vi "Main.vi"() -> ()   [LabVIEW 2013]
doc: "This sample project is built upon the standard state machine template and shows how you could create an application that acquires, analyzes, and presents data. It includes functionality for presenting configuration dialogs, preserving settings between executions, loading and saving data, as well as exporting graph images and text files.\n\nIt is most appropriate for data that is acquired instantly as it does not allow for screen updates mid acquisition nor does it allow for continuous streaming to disk."
uses:
  TimeTagLV.lvlib
panel:
  in  "Record data":bool
  out "Initial time":dbl
  out "Elapsed time (s)":dbl
  out "FPGA_Run Status":dbl
  out "USB_Open Status":dbl
  out "Channel 4 Total\nCounts":dbl
  out "Channel 3 Total\nCounts":dbl
  out "Channel 2 Total\nCounts":dbl
  out "Channel 1 Total\nCounts":dbl
  in  "File Name":string
  out "?":dbl
  out "?":dbl
  out "?":dbl
  out "?":dbl
  in  "Runs":dbl
  out "stats":i32[](array[numeric])
  in  "stop":bool
  out "Channel 4 CPS":dbl(knob) scale=0.0..10000.0
  out "Channel 3 CPS":dbl(knob) scale=0.0..10000.0
  out "Channel 2 CPS":dbl(knob) scale=0.0..10000.0
  out "Channel 1 CPS":dbl(knob) scale=0.0..10000.0
  # "Channel 1"
  # "Channel 2"
  # "Channel 3"
  # "Channel 4"
  # "Coincidence Channels 1 & 2"
  # "Coincidence Channels 1 & 3"
  # "Coincidence Channels 1 & 4"
  # "Coincidence Channels 2 & 3"
  # "Coincidence Channels 2 & 4"
  # "Coincidence Channels 3 & 4"
  # "Coincidence Channels 1 & 2 & 3"
  # "Coincidence Channels 1 & 2 & 4"
  # "Coincidence Channels 1 & 3 & 4"
  # "Coincidence Channels 2 & 3 & 4"
  # "Coincidence Channels 1 & 2 & 3 & 4"
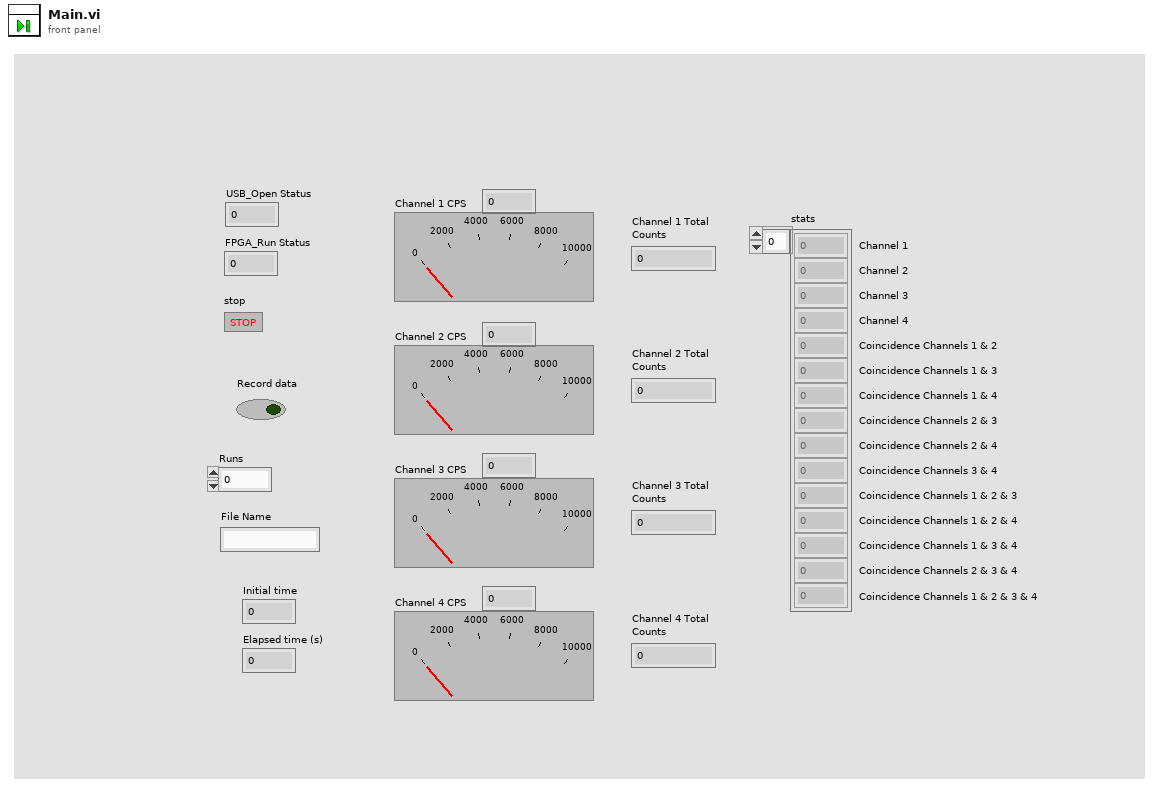
[diagram p1: front panel]
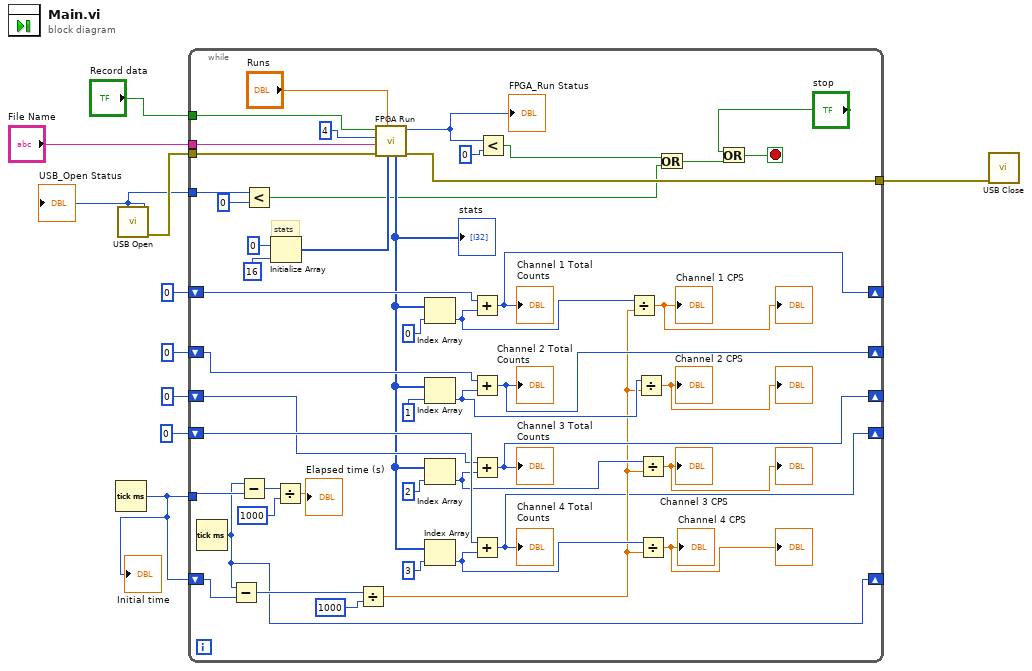
[diagram p0: block diagram]
diagram:
  n1 = Tick Count (ms)() -> (millisecond timer value=w2:u32)
  "Initial time" <- w2
  n2 = call "USB Open.vi"() -> ("error out"=w4:errorcluster, "function return"=w1:i32)  [unwired: 10 in]
  "USB_Open Status" <- w1
  n3 = while {
    tunnel: w2 -> [w58]
    shift-right: [w17] -> _
    shift-left: 0 -> [w48]
    shift-right: [w43] -> _
    shift-left: 0 -> [w49]
    shift-right: [w42] -> _
    shift-left: 0 -> [w50]
    shift-right: [w18] -> _
    shift-left: 0 -> [w51]
    tunnel: w4 -> [w33]
    tunnel: [w34] -> w3
    tunnel: "Record data" -> [w30]
    tunnel: "File Name" -> [w31]
    shift-right: [w16] -> _
    shift-left: w2 -> [w26]
    tunnel: w1 -> [w14]
    stop <- w40 stop-if-true
    # "stats"
    n4 = Tick Count (ms)() -> (millisecond timer value=w16:u32)
    n5 = Subtract(x=w16, y=w26) -> (x-y=w21:u32)
    n6 = Subtract(x=w16, y=w58) -> (x-y=w57:u32)
    n7 = Less?(x=w14, y=0) -> (x < y?=w12:bool)
    n8 = Initialize Array(0, 16) -> (w36:i32[])
    n9 = Divide(x=w57, y=1000) -> (x/y=→"Elapsed time (s)":dbl)
    n10 = Divide(x=w21, y=1000) -> (x/y=w19:dbl)
    n11 = call "FPGA Run.vi"("stats"=w36, "runs"="Runs", "error in (no error)"=w33, "fileName"=w31, "fpgaCommand"=4, "saveClicks"=w30) -> ("error out"=w34:errorcluster, "function return"=w28:i32, "stats out"=w35:i32[])  [unwired: 3 in]
    "stats" <- w35
    "FPGA_Run Status" <- w28
    n12 = Index Array(array=w35, index=0) -> (element=w25:i32)
    n13 = Index Array(array=w35, index=1) -> (element=w24:i32)
    n14 = Index Array(array=w35, index=2) -> (element=w23:i32)
    n15 = Index Array(array=w35, index=3) -> (element=w22:i32)
    n16 = Add(x=w48, y=w25) -> (x+y=w17:i32)
    "Channel 1 Total\nCounts" <- w17
    n17 = Add(x=w49, y=w24) -> (x+y=w43:i32)
    "Channel 2 Total\nCounts" <- w43
    n18 = Add(x=w50, y=w23) -> (x+y=w42:i32)
    "Channel 3 Total\nCounts" <- w42
    n19 = Add(x=w51, y=w22) -> (x+y=w18:i32)
    "Channel 4 Total\nCounts" <- w18
    n20 = Less?(x=w28, y=0) -> (x < y?=w13:bool)
    n21 = Divide(x=w25, y=w19) -> (x/y=→"Channel 1 CPS" →"?":dbl)
    n22 = Divide(x=w24, y=w19) -> (x/y=→"Channel 2 CPS" →"?":dbl)
    n23 = Divide(x=w23, y=w19) -> (x/y=→"Channel 3 CPS" →"?":dbl)
    n24 = Divide(x=w22, y=w19) -> (x/y=→"Channel 4 CPS" →"?":dbl)
    n25 = Or(x=w13, y=w12) -> (x .or. y?=w11:bool)
    n26 = Or(x="stop", y=w11) -> (x .or. y?=w40:bool)
  }
  n27 = call "USB Close.vi"("error in (no error)"=w3) -> ()  [unwired: 9 in, 2 out]
